vi "AO Create Task.vi"(8 "error in":errorcluster, 11 "Config":T1={"AO config"=[], "AI config"=[], "DI config"=[], "DO config"=[], "TC config"=[{"Channel_Name"="", "Channel_Number"="", "Pre_Scale_min"=0.0, "Pre_Scale_max"=0.0, "units"=4, " type"=7}], "ACC config"=[], "SG config"=[], "Strain Gauge Settings"={"poisson ratio"=0.3, "nominal gage resistance"=120.0, "gage factor"=2.08}, "bridge information"={"strain configuration"=10271, "lead wire resistance"=1.7, "initial bridge voltage"=0.0, "voltage excitation source"=10200, "voltage excitation value"=3.3}, "Sample Rate"={"AI Sample Rate"=0.0, "AO Sample Rate"=0.0, "DI Sample Rate"=0.0, "TC Sample Rate"=0.0, "DO Sample Rate"=0.0, "SG Sample Rate"=0.0, "ACC Sample Rate"=0.0}} {"bridge information"."initial bridge voltage" format="%0.2f"; "bridge information"."voltage excitation source" items=["Internal"=10200, "External"=10167, "None"=10230]; "bridge information"."voltage excitation value" format="%0.2f"; "bridge information"."lead wire resistance" format="%0.2f"; "bridge information"."strain configuration" items=["Full Bridge I"=10183, "Full Bridge II"=10184, "Full Bridge III"=10185, "Half Bridge I"=10188, "Half Bridge II"=10189, "Quarter Bridge I"=10271, "Quarter Bridge II"=10272]; "ACC config"."Terminal configuration" items=["default"=-1, "RSE"=10083, "NRSE"=10078, "Differential"=10106, "Pseudodifferential"=12529]; "ACC config"."Sensitivity units" items=["mVolts/g"=12509, "Volts/g"=12510]; "TC config"."type" items=["J"=10072, "K"=10073, "N"=10077, "R"=10082, "S"=10085, "T"=10086, "B"=10047, "E"=10055]; "TC config"."units" items=["Deg C", "Deg F", "Kelvins", "Deg R", "From Custom Scale"]}) -> (0 "error out":errorcluster, 2 "empty?":bool, 3 "task out":refnum<k21>)   [LabVIEW 2022 SP3]
uses:
  Controls/Config.ctl
  <vilib>/DAQmx/create/channels.llb/DAQmx Create Channel (AO-Voltage-Basic).vi
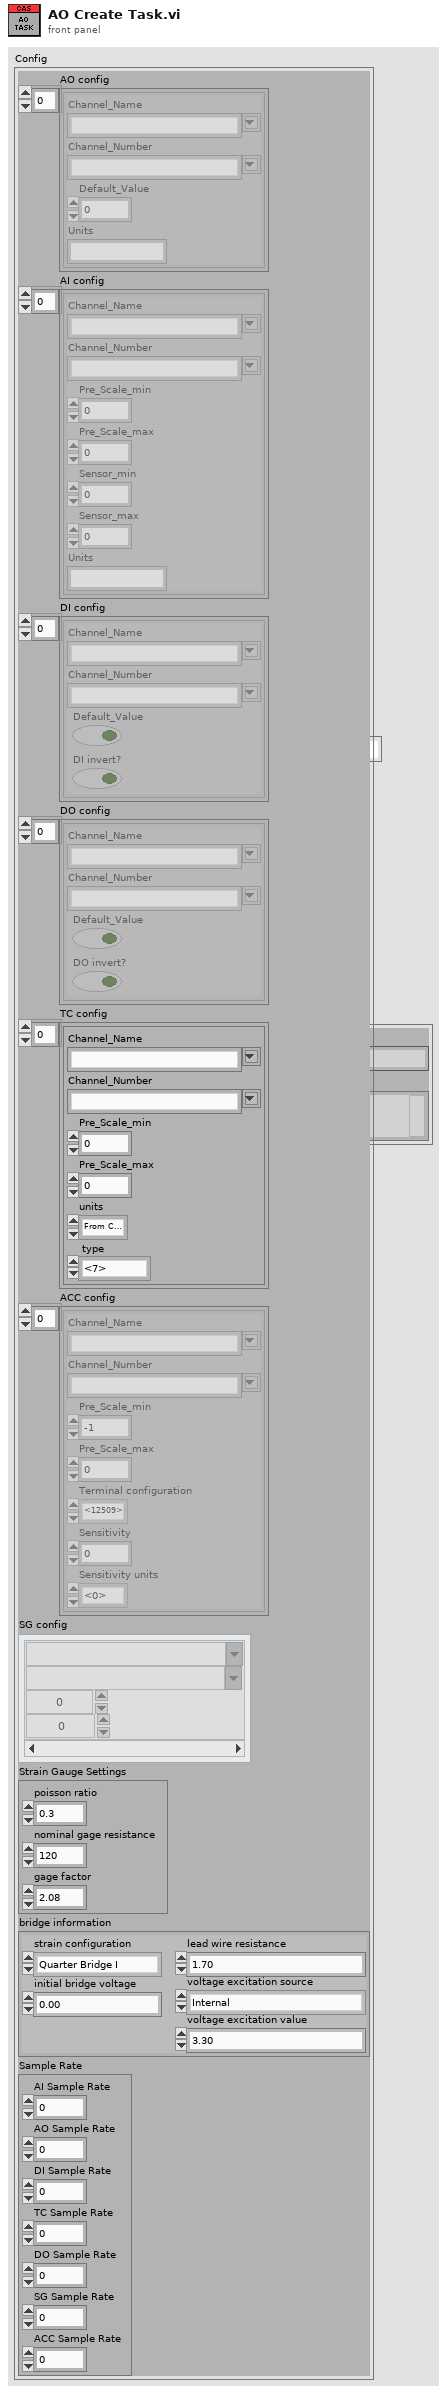
[diagram p1: front panel]
types:
  T1 = typedef "Config.ctl" = cluster{"AO config":cluster{"Channel_Name":string, "Channel_Number":string, "Default_Value":dbl, "Units":string}[], "AI config":cluster{"Channel_Name":string, "Channel_Number":string, "Pre_Scale_min":dbl, "Pre_Scale_max":dbl, "Sensor_min":dbl, "Sensor_max":dbl, "Units":string}[], "DI config":cluster{"Channel_Name":string, "Channel_Number":string, "Default_Value":bool, "DI invert?":bool}[], "DO config":cluster{"Channel_Name":string, "Channel_Number":string, "Default_Value":bool, "DO invert?":bool}[], "TC config":cluster{"Channel_Name":string, "Channel_Number":string, "Pre_Scale_min":dbl, "Pre_Scale_max":dbl, "units":i32, " type":i32}[], "ACC config":cluster{"Channel_Name":string, "Channel_Number":string, "Pre_Scale_min":dbl, "Pre_Scale_max":dbl, "Terminal configuration":i32, "Sensitivity":dbl, "Sensitivity units":i32}[], "SG config":cluster{"Channel_Name":string, "Channel_Number":string, "Pre_Scale_min":dbl, "Pre_Scale_max":dbl}[], "Strain Gauge Settings":cluster{"poisson ratio":dbl, "nominal gage resistance":dbl, "gage factor":dbl}, "bridge information":cluster{"strain configuration":i32, "lead wire resistance":dbl, "initial bridge voltage":dbl, "voltage excitation source":i32, "voltage excitation value":dbl}, "Sample Rate":cluster{"AI Sample Rate":dbl, "AO Sample Rate":dbl, "DI Sample Rate":dbl, "TC Sample Rate":dbl, "DO Sample Rate":dbl, "SG Sample Rate":dbl, "ACC Sample Rate":dbl}}
  T2 = cluster{"Channel_Name":string, "Channel_Number":string, "Default_Value":dbl, "Units":string}[]
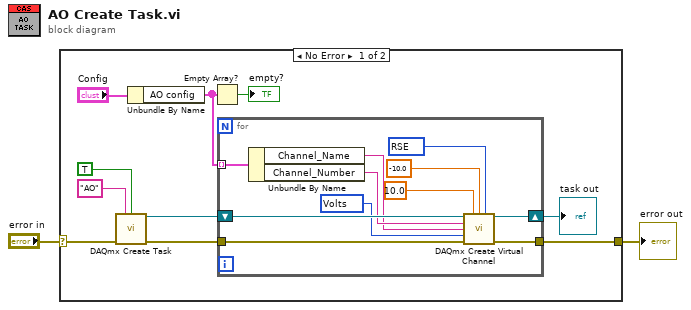
[diagram p0: block diagram]
diagram:
  n1 = case shown="No Error" "error in" {
    selector: "error in" -> [w9 w24]
    tunnel: [w6 w24] -> w1
    frame No Error {
      n2 = call <vilib>:"DAQmx Create Task.vi"("new task name"="AO", "auto cleanup"=TRUE, "error in"=w9) -> ("task out"=w10:refnum<k21>, "error out"=w12:errorcluster)  [unwired: 11 in]
      n3 = Unbundle By Name("Config") -> ("AO config"=w3:T2)
      n4 = Empty Array?(array=w3) -> (empty?=→"empty?":bool)
      n5 = for {
        tunnel: w3 -> [w19] mode=indexing
        tunnel: w12 -> [w21]
        tunnel: [w20] -> w6
        shift-right: [w22] -> w7
        shift-left: w10 -> [w23]
        w14 = 10083 items=["Default"=-1, "RSE"=10083, "Differential"=10106, "Pseudodifferential"=12529] ("output terminal configuration")
        w17 = 10348 items=["Volts"=10348, "From Custom Scale"=10065] ("units")
        n6 = Unbundle By Name(w19) -> ("Channel_Name"=w13:string, "Channel_Number"=w18:string)
        n7 = call-poly <vilib>:"DAQmx Create Virtual Channel.vi"("task in"=w23, "maximum value"=10.0, "minimum value"=-10.0, "output terminal configuration"=w14, "physical channels"=w18, "name to assign"=w13, "units"=w17, "error in"=w21) -> ("task out"=w22:refnum<k21>, "error out"=w20:errorcluster)  [unwired: 6 in]
      }
      "task out" <- w7
    }
    frame Error {
    }
  }
  "error out" <- w1
